vi "PID no reset.vi"(4 "State":i16, 5 "Time":dbl format="%.2f", 6 "Sensor Values":dbl[](array[numeric]), 7 "Set Points":dbl[](array[numeric])) -> (0 "required data":T1={"Set Point names"=["target value", "P Kc", "I Ti (min)", "D Td (min)"], "required number of setpoints"=4, "required number of sensors"=1, "Sensor names"=["Measured process value"]}, 3 "output value":dbl)   [LabVIEW 2012]
uses:
  PID library.llb/PID.vi
  PID library.llb/PID (DBL).vi
panel:
  # "Enter the correct information for this control code in the required data structure below. Then make the current value default by right clicking on the border of the data structure."
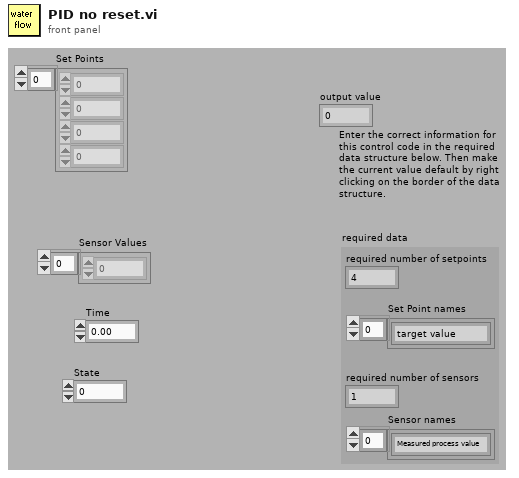
[diagram p1: front panel]
types:
  T1 = cluster{"Set Point names":string[], "required number of setpoints":u8, "required number of sensors":u8, "Sensor names":string[]}
  T2 = cluster{"Set Points[0]":dbl, "Set Points[1]":dbl, "Set Points[2]":dbl, "Set Points[3]":dbl}
  T3 = cluster{"Set Points[1]":dbl, "Set Points[2]":dbl, "Set Points[3]":dbl}
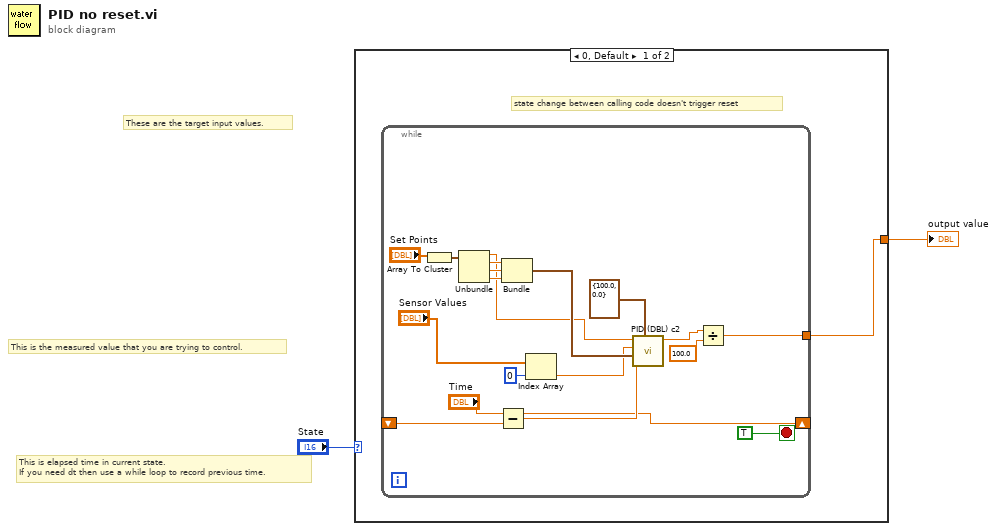
[diagram p0: block diagram]
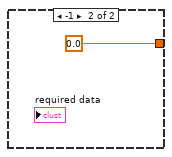
[diagram p2: hidden frame]
diagram:
  # "These are the target input values."
  # "This is the measured value that you are trying to control."
  # "This is elapsed time in current state.\nIf you need dt then use a while loop to record previous time."
  n1 = case shown="0, Default" "State" {
    tunnel: [w3 0.0 ("fraction on")] -> w2
    frame 0, Default {
      # "state change between calling code doesn't trigger reset"
      n2 = while {
        shift-right: ["Time"] -> _
        shift-left: _ -> [w20]
        tunnel: [w13] -> w3
        stop <- TRUE stop-if-true
        n3 = Array To Cluster(array="Set Points") -> (cluster=w12:T2)
        n4 = Unbundle(w12) -> ("Set Points[0]"=w4:dbl, "Set Points[1]"=w10:dbl, "Set Points[2]"=w11:dbl, "Set Points[3]"=w9:dbl)
        n5 = Subtract(x="Time", y=w20) -> (x-y=w19:dbl)
        n6 = Bundle("Set Points[1]"=w10, "Set Points[2]"=w11, "Set Points[3]"=w9) -> (w8:T3)  [unwired: 1 in]
        n7 = Index Array(array="Sensor Values", index=0) -> (element=w5:dbl)
        n8 = call-poly "PID (DBL) c2.vi"("output range"=cluster{"output high":dbl, "output low":dbl} {"output high"=100.0, "output low"=0.0}, "dt (s)"=w19, "PID gains"=w8, "process variable"=w5, "setpoint"=w4) -> ("output"=w17:dbl)  [unwired: 5 in, 1 out]
        n9 = Divide(x=w17, y=100.0) -> (x/y=w13:dbl)
      }
    }
    frame -1 {
    }
  }
  "output value" <- w2
